vi "String Not Included.vi"(9 "haystack":string, 10 "needle":string) -> (0 "error out":errorcluster)   [LabVIEW 2017, in "Transparent Assertions.Tests.lvlib" / "Assert String Not Contains String.lvlib"]
uses:
  Assert String Not Contains String.lvlib
  src/Transparent Assertions/Transparent Assertions.lvlib
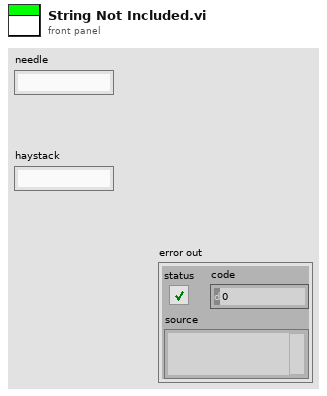
[diagram p1: front panel]
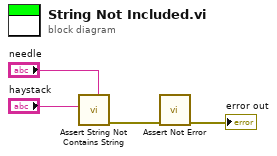
[diagram p0: block diagram]
diagram:
  n1 = call "Assert String Not Contains String.vi"("Needle"="needle", "Haystack"="haystack") -> ("error out"=w1:errorcluster)  [unwired: 9 in]
  n2 = call "Assert Not Error.vi"("error in (no error)"=w1) -> ("error out"=→"error out":errorcluster)  [unwired: 10 in]
